vi "Coins.vi"(8 "error in (no error)":errorcluster, 10 "Coins":cluster{"1":bool, "2":bool, "5":bool}, 11 "Monedas MXN in":refnum<class "Monedas MXN.lvclass">) -> (0 "error out":errorcluster, 3 "Monedas MXN out":refnum<class "Monedas MXN.lvclass">)   [LabVIEW 2020, in "Monedas MXN.lvlib" / "Monedas MXN.lvclass"]
uses:
  Monedas MXN.lvclass
  C:/Program Files (x86)/National Instruments/LabVIEW 2020/vi.lib/ActorFramework/Actor/Actor.lvclass
  <vilib>/ActorFramework/Actor/Actor.lvclass/Actor.ctl
  Monedas MXN.lvclass/Monedas MXN.ctl
  UI Actor Messages/Add credit Msg/Add credit Msg.lvclass/Add credit Msg.ctl
  <vilib>/ActorFramework/Message Enqueuer/Message Enqueuer.lvclass/Message Enqueuer.ctl
  <vilib>/ActorFramework/Message Enqueuer/Enqueue.vi
  UI Actor Messages/Add credit Msg/Add credit Msg.lvclass
  C:/Program Files (x86)/National Instruments/LabVIEW 2020/vi.lib/ActorFramework/Message/Message.lvclass
  <vilib>/ActorFramework/Message Priority Queue/Priority Enqueue.vi
  <vilib>/ActorFramework/Actor/Actor.lvclass
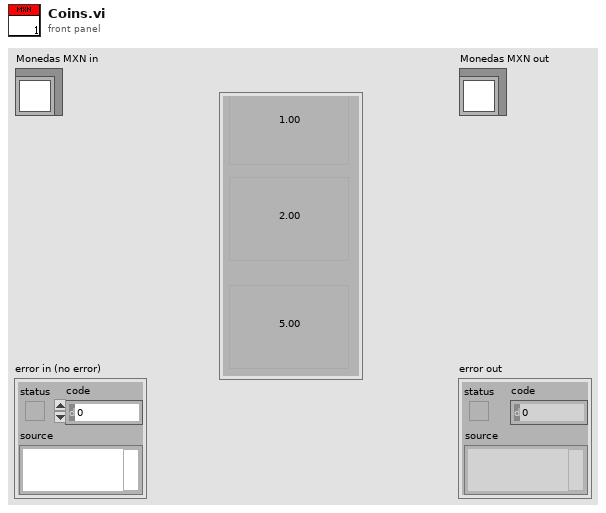
[diagram p1: front panel]
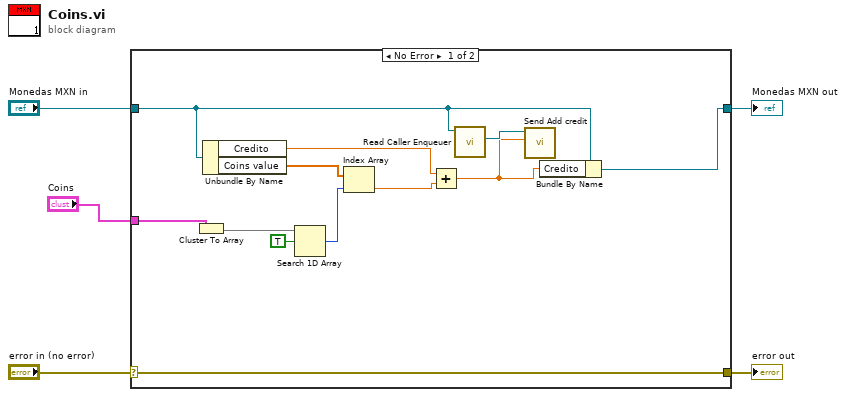
[diagram p0: block diagram]
diagram:
  n1 = case shown="No Error" "error in (no error)" {
    selector: "error in (no error)" -> [w17 w19]
    tunnel: [w17 w19] -> w4
    tunnel: [w9 w18] -> w2
    tunnel: "Monedas MXN in" -> [w8 w18]
    tunnel: "Coins" -> [w16 _]
    frame No Error {
      n2 = Cluster To Array(cluster=w16) -> (array=w15:bool[])
      n3 = Unbundle By Name(w8) -> ("Credito"=w10:dbl, "Coins value"=w13:dbl[])
      n4 = Search 1D Array(1D array=w15, element=TRUE) -> (index of element=w12:i32)  [unwired: 1 in]
      n5 = Index Array(array=w13, index=w12) -> (element=w11:dbl)
      n6 = Add(x=w10, y=w11) -> (x+y=w6:dbl)
      n7 = call <vilib>:"Read Caller Enqueuer.vi"("Actor"=w8) -> ("Caller Enqueuer"=w7:refnum<class "Message Enqueuer.lvclass">)  [unwired: 10 in]
      n8 = call "Send Add credit.vi"("Credito"=w6, "Message Enqueuer"=w7) -> ()  [unwired: 8 in, 2 out]
      n9 = Bundle By Name(cluster=w8, "Credito"=w6) -> (w9:refnum<class "Monedas MXN.lvclass">)
    }
    frame Error {
    }
  }
  "error out" <- w4
  "Monedas MXN out" <- w2
